vi "Exit TestMode.vi"(8 "error in (no error)":errorcluster caption="错误输入（无错误）") -> (0 "error out":errorcluster caption="错误输出")   [LabVIEW 2024]
uses:
  Ctrl/PLC Enum.ctl
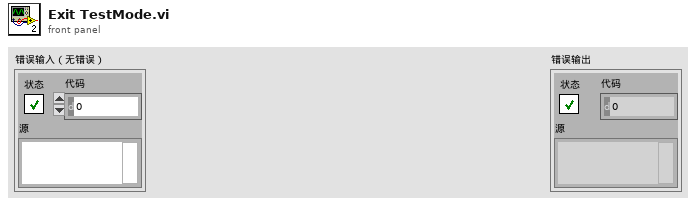
[diagram p1: front panel]
types:
  T1 = typedef "PLC Enum.ctl" = enum16{"Init", "Enable", "Orign", "Load", "Start", "Stop", "StartTest", "StopTest", "Reflector", "WriteResult", "SetSpeed", "SetOrign", "SetLoad", "ServoStatus?", "EquipStatus?", "Origin?", "TestStatus?", "Loadstatus?", "DUTStatus?", "Mes?", "Error？", "Position？", "Speed?", "PinCount", "RunMode", "SN", "Reset", "Jog+", "Jog-", "Close", "Up", "Down", "Clamp", "Release", "In", "Out", "EnterTestMode", "ExitTestMode", "StartButton", "ScanOK", "Power"}
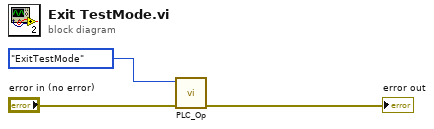
[diagram p0: block diagram]
diagram:
  n1 = call "PLC_Op.vi"("error in (no error)"="error in (no error)", "Status"=PLC_Enum."ExitTestMode") -> ("error out"=→"error out":errorcluster)  [unwired: 4 in, 5 out]
